vi "运维调试_总磷总氮.vi"() -> ()   [LabVIEW 2016, in "斯坦道总氮.lvlib"]
uses:
  <vilib>/Utility/miscctls.llb/LVPointTypeDef.ctl
  <vilib>/Plasmionique/MB Master/MB_Master/MB_Master.lvclass
  <vilib>/ptbypt/NI_PtbyPt.lvlib
  Alarm interface/Alarm interface.lvlib
panel:
  in  "周期设置":bool
  in  "流程操作":bool
  out "消解压力":sgl format="%#.2f kPa"
  out "权限等级":string
  out "总步数":i32
  out "滑动杆":u8(slide) caption="测试进度" scale=0.0..100.0
  in  "关闭心跳包":bool
  out "试剂余量显示":sgl[][](graph)
  in  "仪器校准":bool
  in  "参数查询":bool
  out "简易步骤名称":string
  in  "温度曲线":bool
  in  "试剂余量":bool
  in  "灯值调整":bool
  out "固件版本号":string
  out "模块版本号":string
  out "注射器温度":sgl format="%#.2f ℃"
  out "消解温度":sgl format="%#.2f ℃"
  out "ADC":sgl
  out "F3":sgl format="%#.6f"
  out "F2":sgl format="%#.6f"
  out "F1":sgl format="%#.6f"
  out "F0":sgl format="%#.6f"
  out "运行状态":T1 {"数据时间:" format="%<%y/%m/%d %H:%M:%S>T"; "仪器时间:" format="%<%y/%m/%d %H:%M:%S>T"}
  in  "单选按钮":T2=enum."总氮"
  in  "布尔":bool
  in  "外设固件":bool
  out "字符串 2":string
  in  "数组":string[](array[string])
  in  "返回":bool
  in  "参数设置":bool
  out "集成报警信息":string
  in  "停止":bool
  in  "手动启动":bool
  in  "调试":bool
  out "多列列表框":i32(listbox)
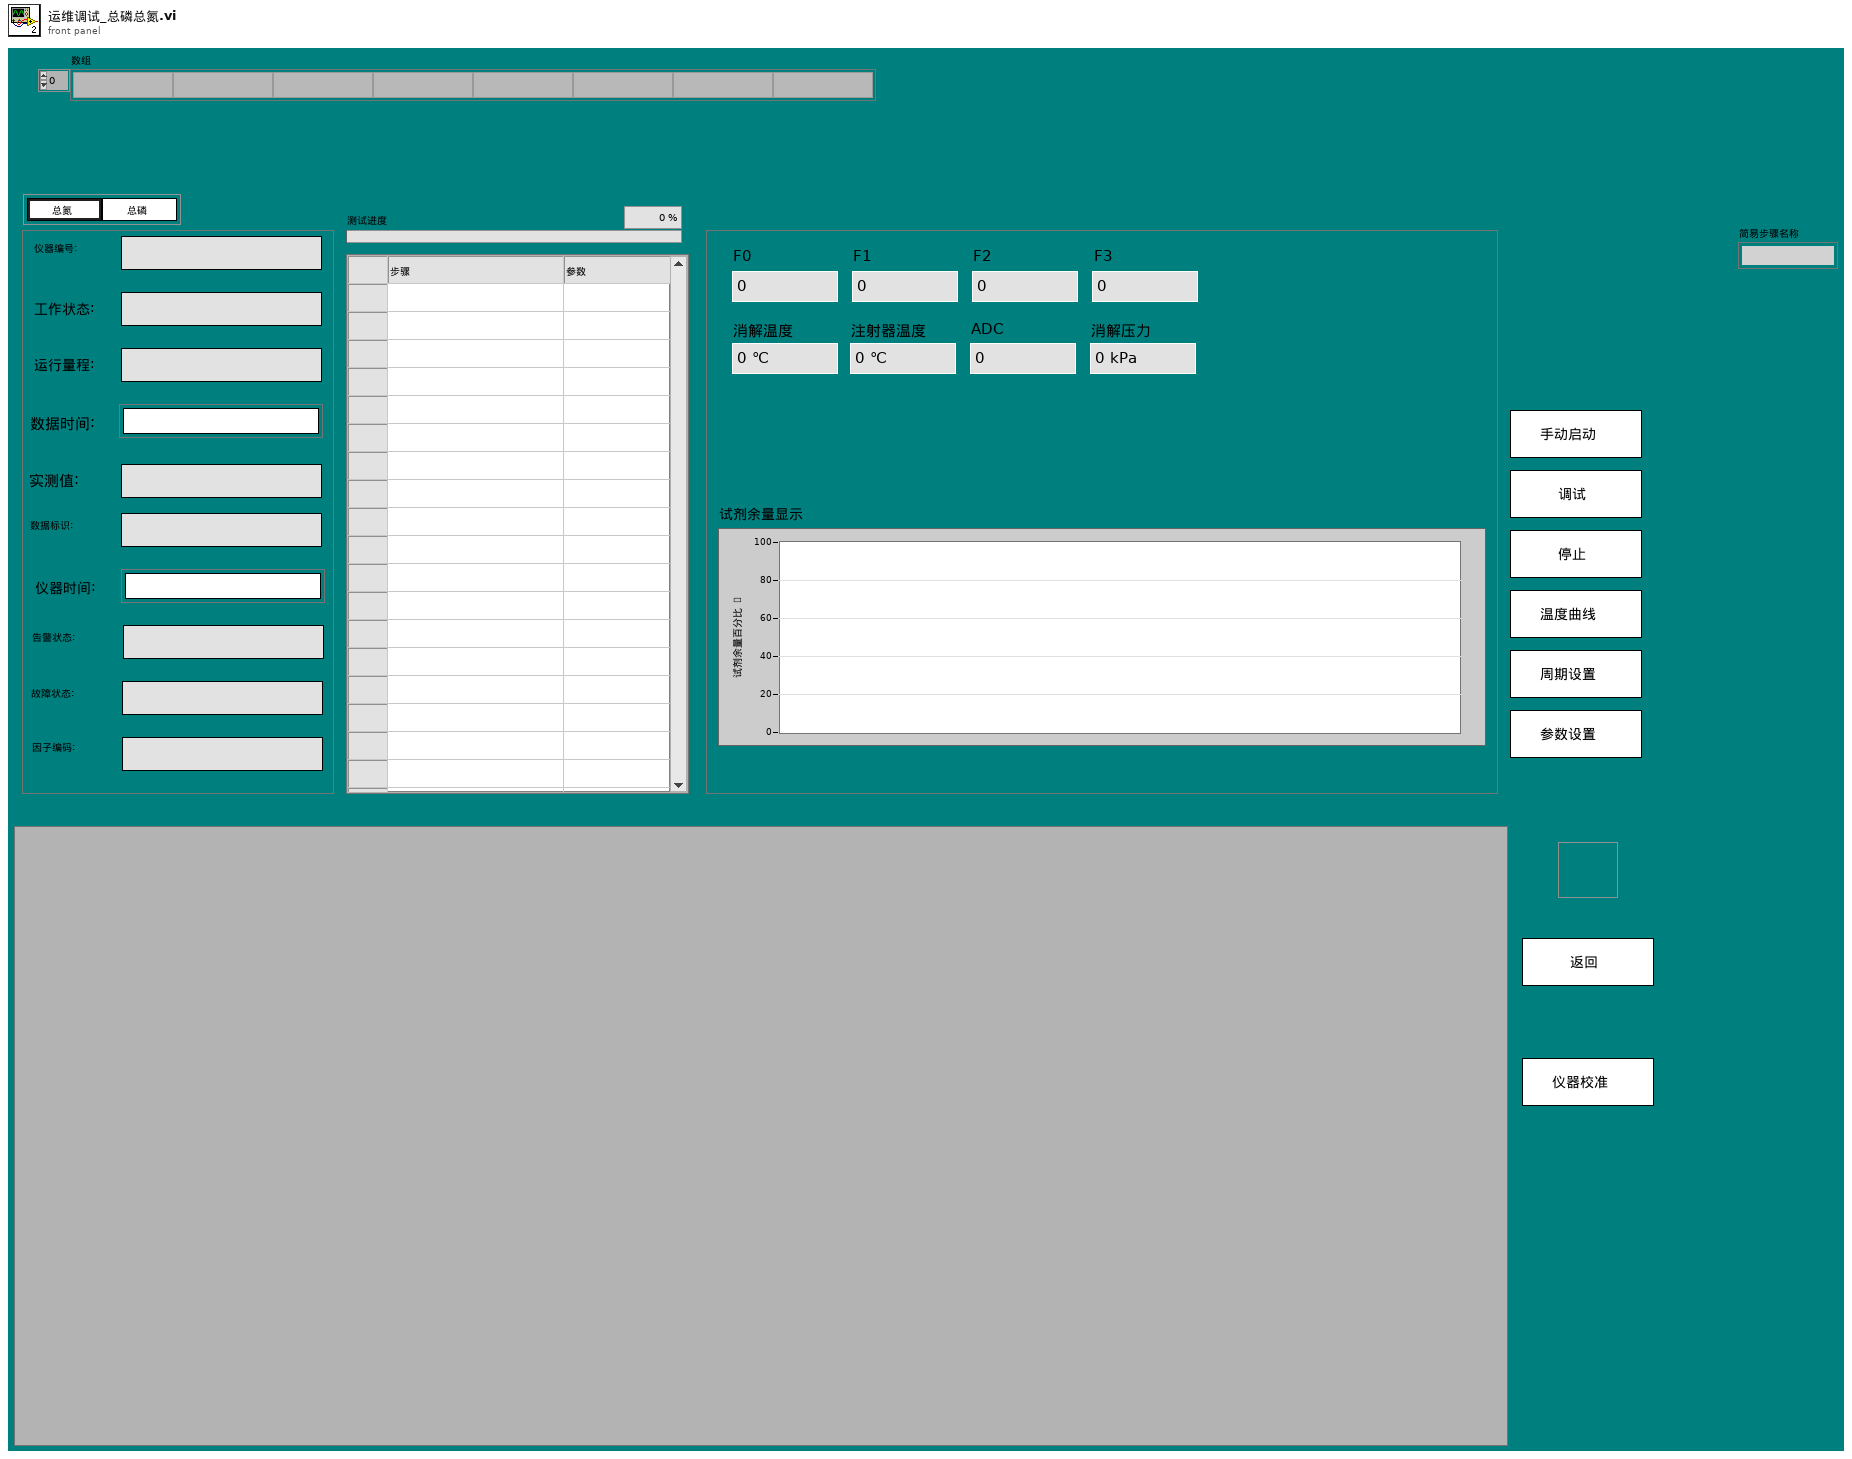
[diagram p1: front panel]
types:
  T1 = cluster{"仪器编号:":string, "工作状态:":string, "运行量程: ":string, "数据时间:":timestamp, "实测值:":string, "数据标识: ":string, "仪器时间:":timestamp, "告警状态: ":string, "故障状态:  ":string, "因子编码:":string}
  T2 = typedef "斯坦道总氮.lvlib/启动参数显示控件.ctl" = enum32{"COD", "氨氮", "总氮", "总磷", "磷酸盐", "硝氮", "亚硝氮", "硅酸盐", "硫化物", "氟化物"}
  T3 = cluster{"Major":u16, "Minor":u16, "Fix":u16, "Build":u16}
  T4 = enum32{"COD", "氨氮", "总氮", "总磷", "磷酸盐", "硝氮", "亚硝氮", "硅酸盐", "硫化物", "氟化物"}
  T5 = typedef "LVPointTypeDef.ctl" = cluster{"Horizontal":i16, "Vertical":i16}
  T6 = cluster{"系统时间":timestamp, "工作状态":u16, "测量模式":enum16{"待机", "连续模式", "周期模式", "定点模式", "受控模式", "手动模式"}, "告警代码":u16, "故障代码":u16, "日志代码":u16, "软件版本":u16, "F0":sgl, "F1":sgl, "F2":sgl, "F3":sgl, "T":sgl, "H":sgl, "id":u16, "flowid":u16, "量程":u16, "总磷控温温度1":sgl, "营养盐控温温度2":sgl, "ADC":sgl}
  T7 = cluster{"modid":i32, "sysid":i32, "content":string, "故障详情":string}
  T8 = typedef "SingleStepTestV3.lvlib/SingleStepTestV3.lvclass/仪器版本.ctl" = enum16{"A版", "B版"}
  T9 = cluster{"因子编码":u32, "单位":u16, "标样参考值":sgl, "水样数据时间":timestamp, "水样实测值":sgl, "水样数据标识":string, "标样数据时间":timestamp, "标样实测值":sgl, "标样数据标识":string, "空白数据时间":timestamp, "空白实测值":sgl, "空白数据标识":string, "零点核查数据时间":timestamp, "零点核查实测值":sgl, "零点核查数据标识":string, "跨度核查数据时间":timestamp, "跨度核查实测值":sgl, "跨度核查数据标识":string, "加标回收数据时间":timestamp, "加标回收实测值":sgl, "加标回收数据标识":string, "平行样数据时间":timestamp, "平行样实测值":sgl, "平行样数据标识":string, "F0":sgl, "F1":sgl, "F2":sgl, "F3":sgl, "F4":sgl, "F5":sgl, "F6":sgl, "F7":sgl, "温度":sgl, "湿度":sgl, "X值":sgl, "fidrange":u16, "X1值":sgl}[]
  T10 = cluster{"因子编码":u32, "单位":u16, "标样参考值":sgl, "水样数据时间":timestamp, "水样实测值":sgl, "水样数据标识":string, "标样数据时间":timestamp, "标样实测值":sgl, "标样数据标识":string, "空白数据时间":timestamp, "空白实测值":sgl, "空白数据标识":string, "零点核查数据时间":timestamp, "零点核查实测值":sgl, "零点核查数据标识":string, "跨度核查数据时间":timestamp, "跨度核查实测值":sgl, "跨度核查数据标识":string, "加标回收数据时间":timestamp, "加标回收实测值":sgl, "加标回收数据标识":string, "平行样数据时间":timestamp, "平行样实测值":sgl, "平行样数据标识":string, "F0":sgl, "F1":sgl, "F2":sgl, "F3":sgl, "F4":sgl, "F5":sgl, "F6":sgl, "F7":sgl, "温度":sgl, "湿度":sgl, "X值":sgl, "fidrange":u16, "X1值":sgl}
  T11 = typedef "报警信息字段定义.ctl" = cluster{"时间":timestamp, "参数":string, "报警信息":string, "备注":string, "code":u64}
  T12 = cluster{"module name":string, "moduleid":i32, "sysid":i32, "content":string, "analysis":string}
  T13 = cluster{"参数":string, "报警内容":string, "报警分析":string}
  T14 = typedef "TimingControl.lvlib/TimingControl.lvclass/国标控制命令.ctl" = enum16{"启动测量", "标样核查", "零点核查", "跨度核查", "空白测试", "平行样测试", "加标回收", "空白校准", "标样校准", "初始化（清洗）", "停止测试", "仪器重启", "校时", "模式设置", "测量间隔设置"}
  T15 = typedef "TimingControl.lvlib/TimingControl.lvclass/测量参数.ctl" = u16
  T16 = enum32{"Bad", "Idle", "Run top level", "Running"}
  T17 = enum16{"空闲", "水样测试", "标样核查", "零点核查", "跨度核查", "空白测试", "平行样测试", "加标回收", "空白校准", "标样校准", "初始化（清洗）"}
  T18 = cluster{"站号":u16, "量程切换":enum32{"H", "L", "AUTO"}, "控制命令":enum16{"启动测量", "标样核查", "零点核查", "跨度核查", "空白测试", "平行样测试", "加标回收", "空白校准", "标样校准", "初始化（清洗）", "停止测试", "仪器重启", "校时", "模式设置", "测量间隔设置"}, "模式设置":enum16{"待机", "连续模式", "周期模式", "定点模式", "受控模式", "手动模式"}, "测量间隔":u16}
  T19 = cluster{"时间标识":timestamp, "设备":string, "日志信息":string, "流程参数":string}
  T20 = typedef "LVRowAndColumnUnsignedTypeDef.ctl" = cluster{"Row":u32, "Column":u32}
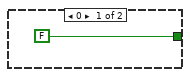
[diagram p4: hidden frame]
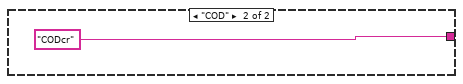
[diagram p5: hidden frame]
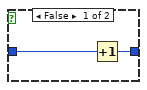
[diagram p7: hidden frame]
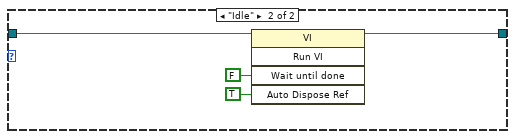
[diagram p8: hidden frame]
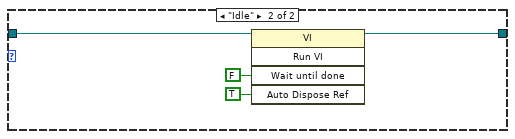
[diagram p9: hidden frame]
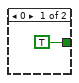
[diagram p11: hidden frame]
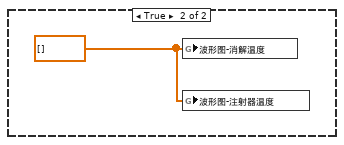
[diagram p12: hidden frame]
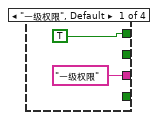
[diagram p16: hidden frame]
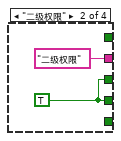
[diagram p17: hidden frame]
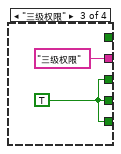
[diagram p18: hidden frame]
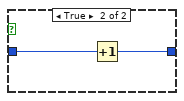
[diagram p20: hidden frame]
diagram:
  n1 = flat-sequence {
    tunnel: [w29] -> w20
    tunnel: [w31] -> w18
    tunnel: [w30] -> w2
    tunnel: w20 -> [w42]
    tunnel: [w42] -> w19
    tunnel: w18 -> [_]
    tunnel: w2 -> [_]
    tunnel: w19 -> [w65]
    tunnel: [w154] -> w21
    tunnel: [errorcluster {"status"=FALSE, "code"=0, "source"=""} ("错误输入（无错误）")] -> w9
    tunnel: [errorcluster {"status"=FALSE, "code"=0, "source"=""} ("错误输入（无错误）")] -> w8
    tunnel: [w151] -> w6
    tunnel: [errorcluster {"status"=FALSE, "code"=0, "source"=""} ("error out")] -> w5
    tunnel: [errorcluster {"status"=FALSE, "code"=0, "source"=""} ("错误输入（无错误）")] -> w4
    frame #0 {
      n2 = control-ref of="本VI"() -> (w32:refnum<vi>)
      n3 = control-ref of="本VI"() -> (w41:refnum<vi>)
      n4 = call "仪器配置读取.vi"() -> ("error out"=w31:errorcluster)  [unwired: 11 in]
      n5 = call "模块配置读取.vi"() -> ("error out"=w30:errorcluster)  [unwired: 11 in]
      n6 = property class="VI"(reference=w32) -> ("Library"=w33:refnum<vi>)  [unwired: 1 in, 2 out]
      n7 = property class="VI"(reference=w41) -> ("Library.Version"=w40:T3)  [unwired: 1 in, 2 out]
      n8 = property class="Library"(reference=w33) -> ("LocalName"=w29:string)  [unwired: 1 in, 2 out]
      n9 = Unbundle By Name(w40) -> ("Major"=w38:u16, "Minor"=w37:u16, "Fix"=w36:u16, "Build"=w35:u16)
      n10 = Format Into String(format string="模块版本号：%d.%d.%d.%d" ("格式字符串"), w38, w37, w36, w35) -> (resulting string=→"模块版本号":string)  [unwired: 2 in, 1 out]
    }
    frame #1 {
      n11 = global read "总磷总氮断电保存全局变量.vi" "IP"() -> (w46:string)
      n12 = global read "总磷总氮断电保存全局变量.vi" "VISA Resource"() -> (w43:refnum<visa-resource-name>)
      n13 = Empty String/Path?(string/path=w46) -> (empty?=w45:bool)
      n14 = Empty String/Path?(string/path=w43) -> (empty?=w44:bool)
      n15 = case shown="真" w45 {
        tunnel: w42 -> [_ w57]
        frame False {
        }
        frame True {
          n16 = case shown="\"斯坦道总氮.lvlib\"" w57 {
            tunnel: [w58 "192.168.1.203" ("IP") "192.168.1.202" ("IP") "192.168.1.202" ("IP") "192.168.1.203" ("IP") "192.168.1.204" ("IP") "192.168.1.205" ("IP")] -> w56
            frame Default {
              n17 = global read "总磷总氮断电保存全局变量.vi" "IP"() -> (w58:string)
            }
            frame "斯坦道总磷总氮.lvlib" {
            }
            frame "斯坦道氨氮.lvlib" {
            }
            frame "斯坦道氨氮总磷.lvlib" {
            }
            frame "斯坦道总磷.lvlib" {
            }
            frame "斯坦道总氮.lvlib" {
            }
            frame "斯坦道CODcr.lvlib" {
            }
          }
          n18 = global write "总磷总氮断电保存全局变量.vi" "IP"(w56) -> ()
        }
      }
      n19 = case shown="真" w44 {
        tunnel: w42 -> [_ w48]
        frame False {
        }
        frame True {
          n20 = case shown="\"斯坦道总氮.lvlib\"" w48 {
            tunnel: [w49 "COM5" ("IP") "COM7" ("IP") "COM7" ("IP") "COM5" ("IP") "COM10" ("IP") "COM9" ("IP")] -> w47
            frame Default {
              n21 = global read "总磷总氮断电保存全局变量.vi" "VISA Resource"() -> (w49:refnum<visa-resource-name>)
            }
            frame "斯坦道总磷总氮.lvlib" {
            }
            frame "斯坦道氨氮.lvlib" {
            }
            frame "斯坦道氨氮总磷.lvlib" {
            }
            frame "斯坦道总磷.lvlib" {
            }
            frame "斯坦道总氮.lvlib" {
            }
            frame "斯坦道CODcr.lvlib" {
            }
          }
          n22 = global write "总磷总氮断电保存全局变量.vi" "VISA Resource"(w47) -> ()
        }
      }
    }
    frame #2 {
      n23 = global read "model config var.vi" "启动队列名称"() -> (w67:cluster{"String":string, "Value":u16}[])
      n24 = Empty Array?(array=w67) -> (empty?=w66:bool)
      n25 = case shown="真" w66 {
        tunnel: w65 -> [_ w68]
        frame False {
        }
        frame True {
          n26 = global read "总磷总氮断电保存全局变量.vi" "PORT"() -> (w74:string)
          n27 = Decimal String To Number(string=w74) -> (number=w73:i32)  [unwired: 2 in, 1 out]
          n28 = global read "总磷总氮断电保存全局变量.vi" "MB通信方式选择"() -> (w72:enum16{"串口", "TCP"})
          n29 = global read "总磷总氮断电保存全局变量.vi" "VISA Resource"() -> (w71:refnum<visa-resource-name>)
          n30 = global read "总磷总氮断电保存全局变量.vi" "IP"() -> (w75:string)
          n31 = call "获取启动参数.vi"("MB通信方式选择"=w72, "Port (502)"=w73, "IP Address"=w75, "VISA Resource"=w71) -> ("error out"=w70:errorcluster, "数组"=w69:cluster{"String":string, "Value":u16}[])  [unwired: 6 in]
          n32 = flat-sequence {
            tunnel: w70 -> [w77]
            tunnel: w69 -> [w76]
            tunnel: w68 -> [w79]
            frame #0 {
              n33 = case shown="无错误" w77 {
                tunnel: w76 -> [w78 _]
                frame No Error {
                  n34 = global write "model config var.vi" "启动队列名称"(w78) -> ()
                }
                frame Error {
                }
              }
            }
            frame #1 {
              n35 = global read "model config var.vi" "启动队列名称"() -> (w81:cluster{"String":string, "Value":u16}[])
              n36 = Empty Array?(array=w81) -> (empty?=w80:bool)
              n37 = case shown="真" w80 {
                tunnel: w79 -> [_ w82]
                frame False {
                }
                frame True {
                  n38 = case shown="\"氟化物\"" w82 {
                    frame Default {
                    }
                    frame "斯坦道总磷总氮.lvlib" {
                      n39 = global write "model config var.vi" "启动队列名称"(cluster{"String":string, "Value":u16}[] [{"String"="总氮", "Value"=2}, {"String"="总磷", "Value"=1}] ("启动队列名称")) -> ()
                    }
                    frame "斯坦道氨氮.lvlib" {
                      n40 = global write "model config var.vi" "启动队列名称"(cluster{"String":string, "Value":u16}[] [{"String"="氨氮", "Value"=3}] ("启动队列名称")) -> ()
                    }
                    frame "斯坦道氨氮总磷.lvlib" {
                      n41 = global write "model config var.vi" "启动队列名称"(cluster{"String":string, "Value":u16}[] [{"String"="氨氮", "Value"=3}, {"String"="总磷", "Value"=1}] ("启动队列名称")) -> ()
                    }
                    frame "斯坦道总磷.lvlib" {
                      n42 = global write "model config var.vi" "启动队列名称"(cluster{"String":string, "Value":u16}[] [{"String"="总磷", "Value"=1}] ("启动队列名称")) -> ()
                    }
                    frame "斯坦道总氮.lvlib" {
                      n43 = global write "model config var.vi" "启动队列名称"(cluster{"String":string, "Value":u16}[] [{"String"="总氮", "Value"=2}] ("启动队列名称")) -> ()
                    }
                    frame "斯坦道CODcr.lvlib" {
                      n44 = global write "model config var.vi" "启动队列名称"(cluster{"String":string, "Value":u16}[] [{"String"="CODcr", "Value"=22}] ("启动队列名称")) -> ()
                    }
                    frame "氟化物" {
                      n45 = global write "model config var.vi" "启动队列名称"(cluster{"String":string, "Value":u16}[] [{"String"="氟化物", "Value"=50}] ("启动队列名称")) -> ()
                    }
                  }
                }
              }
            }
            frame #2 {
              n46 = call "模块配置写入.vi"() -> ()  [unwired: 11 in, 1 out]
            }
          }
        }
      }
    }
    frame #3 {
      # "初始化"
      n47 = flat-sequence {
        frame #0 {
          n48 = global read "总磷总氮断电保存全局变量.vi" "流程路径"() -> (w97:path)
          n49 = global read "总磷总氮断电保存全局变量.vi" "简易流程路径"() -> (w94:path)
          n50 = call <vilib>:"Check if File or Folder Exists.vi"("path"=w97) -> ("file or folder exists?"=w102:bool)  [unwired: 8 in, 2 out]
          n51 = call <vilib>:"Check if File or Folder Exists.vi"("path"=w94) -> ("file or folder exists?"=w101:bool)  [unwired: 8 in, 2 out]
          n52 = Empty String/Path?(string/path=w97) -> (empty?=w98:bool)
          n53 = Not(x=w102) -> (.not. x?=w100:bool)
          n54 = Empty String/Path?(string/path=w94) -> (empty?=w93:bool)
          n55 = Not(x=w101) -> (.not. x?=w96:bool)
          n56 = Or(x=w98, y=w100) -> (x .or. y?=w99:bool)
          n57 = Or(x=w93, y=w96) -> (x .or. y?=w95:bool)
          n58 = case shown="真" w99 {
            frame False {
            }
            frame True {
              n59 = global read "model config var.vi" "启动队列名称"() -> (w110:cluster{"String":string, "Value":u16}[])
              n60 = for {
                tunnel: w110 -> [w113] mode=indexing
                tunnel: [w112] -> w109 mode=indexing
                n61 = Unbundle By Name(w113) -> ("String"=w112:string)
              }
              n62 = call "获取默认流程路径.vi"("参数"=w109) -> ("路径"=w111:path)  [unwired: 10 in]
              n63 = global write "总磷总氮断电保存全局变量.vi" "流程路径"(w111) -> ()
            }
          }
          n64 = case shown="真" w95 {
            frame False {
            }
            frame True {
              n65 = global read "model config var.vi" "启动队列名称"() -> (w105:cluster{"String":string, "Value":u16}[])
              n66 = for {
                tunnel: w105 -> [w108] mode=indexing
                tunnel: [w107] -> w104 mode=indexing
                n67 = Unbundle By Name(w108) -> ("String"=w107:string)
              }
              n68 = call "获取默认流程路径.vi"("复合步骤"=TRUE, "参数"=w104) -> ("路径"=w106:path)  [unwired: 9 in]
              n69 = global write "总磷总氮断电保存全局变量.vi" "简易流程路径"(w106) -> ()
            }
          }
        }
        frame #1 {
          n70 = call "仪器配置写入.vi"() -> ()  [unwired: 11 in, 1 out]
        }
      }
      n71 = global read "model config var.vi" "启动队列名称"() -> (w90:cluster{"String":string, "Value":u16}[])
      n72 = for {
        tunnel: w90 -> [w117] mode=indexing
        shift-right: [w116] -> w91
        shift-left: "" -> [w114]
        n73 = Unbundle By Name(w117) -> ("String"=w115:string)
        n74 = Concatenate Strings(w114, w115) -> (w116:string)
      }
      n75 = global write "VAR总磷总氮全局变量.vi" "模块名称"(w91) -> ()
    }
    frame #4 {
      n76 = global read "model config var.vi" "启动队列名称"() -> (w120:cluster{"String":string, "Value":u16}[])
      n77 = vi-ref "总磷总氮测量数据储存.vi"() -> (w130:refnum<vi>)
      n78 = vi-ref "总磷总氮通讯.vi"() -> (w122:refnum<vi>)
      n79 = Index Array(array=w120) -> (element=w119:cluster{"String":string, "Value":u16})  [unwired: 1 in]
      n80 = property class="VI"(reference=w130) -> ("Name"=w137:string)  [unwired: 1 in, 2 out]
      n81 = property class="VI"(reference=w122) -> ("Name"=w123:string)  [unwired: 1 in, 2 out]
      n82 = Unbundle By Name(w119) -> ("Value"=w118:u16)
      n83 = case shown="50" w118 {
        tunnel: [w138 启动参数显示控件."总磷" ("单选按钮") 启动参数显示控件."总氮" ("单选按钮") 启动参数显示控件."COD" ("单选按钮") 启动参数显示控件."氨氮" ("单选按钮") 启动参数显示控件."磷酸盐" ("单选按钮") 启动参数显示控件."硝氮" ("单选按钮") 启动参数显示控件."亚硝氮" ("单选按钮") 启动参数显示控件."硅酸盐" ("单选按钮") 启动参数显示控件."硫化物" ("单选按钮") 启动参数显示控件."氟化物" ("单选按钮")] -> w121
        frame 0, Default {
          n84 = property on="单选按钮" class="RadioBtnsControl (严格)"() -> ("Value"=w138:T4)  [unwired: 2 in, 2 out]
        }
        frame 1 {
        }
        frame 2 {
        }
        frame 22 {
        }
        frame 3 {
        }
        frame 4 {
        }
        frame 5 {
        }
        frame 6 {
        }
        frame 7 {
        }
        frame 8 {
        }
        frame 50 {
        }
      }
      n85 = Open VI Reference(type specifier VI Refnum (for type only)=refnum<vi> refnum, vi path=w137, options=128 ("选项")) -> (vi reference=w135:refnum<vi>, error out=w133:errorcluster)  [unwired: 3 in]
      n86 = Open VI Reference(type specifier VI Refnum (for type only)=refnum<vi> refnum, vi path=w123, options=128 ("选项")) -> (vi reference=w125:refnum<vi>, error out=w127:errorcluster)  [unwired: 3 in]
      n87 = call-by-ref "开始异步调用"(reference=w135, error in=w133) -> (reference out=w131:refnum<vi>, error out=w132:errorcluster)  [unwired: 12 in]
      n88 = call-by-ref "开始异步调用"(reference=w125, error in=w127) -> (reference out=w129:refnum<vi>, error out=w128:errorcluster)  [unwired: 12 in]
      n89 = Close Reference(reference=w131, error in (no error)=w132) -> ()  [unwired: 1 out]
      n90 = Close Reference(reference=w129, error in (no error)=w128) -> ()  [unwired: 1 out]
      n91 = property on="单选按钮" class="RadioBtnsControl (严格)"("Value"=w121) -> ()  [unwired: 2 in, 2 out]
    }
    frame #5 {
      n92 = call "配置文件路径.vi"() -> ("appended path"=w151:path)  [unwired: 11 in]
      n93 = call "设置模块队列名.vi"() -> ("Msg"=w154:string)  [unwired: 5 in]
    }
  }
  n94 = flat-sequence {
    frame #0 {
      n95 = property on="窗格" class="Pane"("Origin"=T5 {"Horizontal"=0, "Vertical"=0} ("原点")) -> ()  [unwired: 2 in, 2 out]
    }
  }
  n96 = call "Create balloon 队列.vi"() -> ("队列输出"=w25:refnum<queue>)  [unwired: 11 in]
  n97 = while {
    stop <- FALSE stop-if-true
    n98 = global read "VAR总磷总氮全局变量.vi" "状态告警区"() -> (w160:T6)
    n99 = Unbundle By Name(w160) -> ("工作状态"=w158:u16)
    n100 = Equal To 0?(x=w158) -> (x = 0?=w157:bool)
    n101 = global read "VAR总磷总氮全局变量.vi" "通讯状态"() -> (w161:bool)
    n102 = And(x=w157, y=w161) -> (x .and. y?=w159:bool)
    n103 = call <vilib>:"Boolean Crossing PtByPt.vi"("input"=w159) -> ("crossing"=w156:bool)  [unwired: 2 in]
    n104 = case shown="真" w156 {
      frame False {
      }
      frame True {
        n105 = control-ref of="试剂余量显示"() -> (w164:refnum<vi>)
        n106 = call "试剂余量展示.vi"("波形图 2"=w164) -> ("波形图"=→"试剂余量显示":sgl[][])  [unwired: 10 in]
      }
    }
    n107 = Wait (ms)(milliseconds to wait=u32 1000 ("等待时间（毫秒）")) -> ()  [unwired: 1 out]
  }
  n108 = while {
    shift-right: [w176] -> _
    shift-left: u32 0 ("y") -> [w178]
    stop <- FALSE stop-if-true
    # "密码权限"
    n109 = global read "VAR总磷总氮全局变量.vi" "权限等级"() -> (w173:enum16{"一级权限", "二级权限", "三级权限", "超级权限"})
    n110 = case shown="\"超级权限\"" w173 {
      tunnel: [_ w183 w185 w188] -> w166
      tunnel: [_ _ w185 w188] -> _
      tunnel: [_ w183 w185 w188] -> w172
      tunnel: [_ _ _ TRUE] -> w171
      tunnel: [TRUE _ _ _] -> w169
      tunnel: ["一级权限" "二级权限" "三级权限" "超级权限"] -> w167
      frame "一级权限", Default {
      }
      frame "二级权限" {
        w183 = TRUE
      }
      frame "三级权限" {
        w185 = TRUE
      }
      frame "超级权限" {
        w188 = TRUE
      }
    }
    "权限等级" <- w167
    n111 = case shown="假" "布尔" {
      tunnel: w178 -> [_ w191]
      tunnel: [_ w190] -> w176
      frame False {
      }
      frame True {
        n112 = Increment(x=w191) -> (x+1=w190:u32)
      }
    }
    n113 = Wait (ms)(milliseconds to wait=u32 1000 ("等待时间（毫秒）")) -> ()  [unwired: 1 out]
    n114 = Not(x=w169) -> (.not. x?=w168:bool)
    n115 = property on="关闭心跳包" class="Bool (严格)"("Visible"=w171) -> ()  [unwired: 2 in, 2 out]
    n116 = property on="外设固件" class="Bool"("Visible"=w172) -> ()  [unwired: 2 in, 2 out]
    n117 = property on="流程操作" class="Bool"("Visible"=w166) -> ()  [unwired: 2 in, 2 out]
    n118 = property on="试剂余量" class="Bool"("Visible"=w166) -> ()  [unwired: 2 in, 2 out]
    n119 = property on="灯值调整" class="Bool"("Visible"=w166) -> ()  [unwired: 2 in, 2 out]
    n120 = Greater Or Equal?(x=w176, y=u32 3600) -> (x >= y?=w174:bool)
    n121 = property on="布尔" class="Bool (严格)"("Value"=w168) -> ()  [unwired: 2 in, 2 out]
    n122 = case shown="真" w174 {
      frame False {
      }
      frame True {
        n123 = global write "VAR总磷总氮全局变量.vi" "权限等级"(enum16{"一级权限", "二级权限", "三级权限", "超级权限"}."一级权限" ("权限等级")) -> ()
      }
    }
  }
  n124 = while {
    shift-right: [w202] -> _
    shift-left: u16 1 ("工作状态") -> [w200]
    stop <- FALSE stop-if-true
    (unwired) "注射器温度"
    n125 = global read "VAR总磷总氮全局变量.vi" "状态告警区"() -> (w223:T6)
    n126 = global read "VAR总磷总氮全局变量.vi" "通讯状态"() -> (w234:bool)
    n127 = global write "VAR总磷总氮全局变量.vi" "最近一次工作状态"(w200) -> ()
    n128 = global read "VAR总磷总氮全局变量.vi" "状态告警区"() -> (w232:T6)
    n129 = Unbundle By Name(w223) -> ("id"=w222:u16, "工作状态"=w218:u16)
    n130 = case shown="真" w234 {
      tunnel: ["通讯异常" ("集成报警信息") w340] -> w233
      frame False {
      }
      frame True {
        n131 = global read "VAR总磷总氮全局变量.vi" "状态告警区"() -> (w346:T6)
        n132 = Unbundle By Name(w346) -> ("工作状态"=w345:u16)
        n133 = feedback #1(0) -> (w343:i32)
        n134 = case shown="0" w345 {
          tunnel: w343 -> [_ w348]
          tunnel: [_ w347] -> w341
          frame 0 {
          }
          frame Default {
            n135 = Increment(x=w348) -> (x+1=w347:i32)
          }
        }
        n136 = feedback-in #1(w341) -> ()
        n137 = global read "VAR总磷总氮全局变量.vi" "测量状态"() -> (w339:string)
        n138 = Format Into String(format string="工作计时: %d 秒" ("格式字符串"), initial string=w339, w341) -> (resulting string=w340:string)  [unwired: 1 in, 1 out]
      }
    }
    "集成报警信息" <- w233
    n139 = Unbundle By Name(w232) -> ("flowid"=w199:u16, "系统时间"=w228:timestamp, "工作状态"=w227:u16, "告警代码"=w221:u16, "故障代码"=w220:u16, "量程"=w226:u16)
    n140 = case shown="\"氨氮\"" "单选按钮" {
      tunnel: [22 3 2 1 4 5 6 7 8 50] -> w203
      tunnel: [_ TRUE _ _ _ _ _ _ _ _] -> w194
      frame "COD", Default {
      }
      frame "氨氮" {
      }
      frame "总氮" {
      }
      frame "总磷" {
      }
      frame "磷酸盐" {
      }
      frame "硝氮" {
      }
      frame "亚硝氮" {
      }
      frame "硅酸盐" {
      }
      frame "硫化物" {
      }
      frame "氟化物" {
      }
    }
    n141 = case shown="1, 默认" w218 {
      tunnel: w222 -> [_ w289]
      frame 0 {
      }
      frame 1, Default {
        n142 = case shown="50" w289 {
          tunnel: [w290 启动参数显示控件."总磷" ("单选按钮") 启动参数显示控件."总氮" ("单选按钮") 启动参数显示控件."COD" ("单选按钮") 启动参数显示控件."氨氮" ("单选按钮") 启动参数显示控件."磷酸盐" ("单选按钮") 启动参数显示控件."硝氮" ("单选按钮") 启动参数显示控件."亚硝氮" ("单选按钮") 启动参数显示控件."硅酸盐" ("单选按钮") 启动参数显示控件."硫化物" ("单选按钮") 启动参数显示控件."氟化物" ("单选按钮")] -> w288
          frame 0, Default {
            n143 = property on="单选按钮" class="RadioBtnsControl (严格)"() -> ("Value"=w290:T4)  [unwired: 2 in, 2 out]
          }
          frame 1 {
          }
          frame 2 {
          }
          frame 22 {
          }
          frame 3 {
          }
          frame 4 {
          }
          frame 5 {
          }
          frame 6 {
          }
          frame 7 {
          }
          frame 8 {
          }
          frame 50 {
          }
        }
        n144 = property on="单选按钮" class="RadioBtnsControl (严格)"("Value"=w288) -> ()  [unwired: 2 in, 2 out]
      }
    }
    n145 = case shown="1" w227 {
      selector: w227 -> [w305 _ w311 w315 w318 w320 w322 w324 w326 w328 w330 w332 w334 w337]
      tunnel: [w306 "空闲" ("工作状态") "水样测量" ("工作状态") w314 "零点核查" ("工作状态") "跨度核查" ("工作状态") "空白测试" ("工作状态") "平行样测试" ("工作状态") "加标回收" ("工作状态") "空白校准" ("工作状态") "标样校准" ("工作状态") "初始化" ("工作状态") "单步调试" ("工作状态") w336] -> w201
      tunnel: [w304 w309 w311 w315 w318 w320 w322 w324 w326 w328 w330 w332 w334 w337] -> w202
      tunnel: w200 -> [w304 w309 _ _ _ _ _ _ _ _ _ _ _ _]
      tunnel: w199 -> [_ _ _ w313 _ _ _ _ _ _ _ _ _ _]
      frame Default {
        n146 = Format Into String(format string="%d" ("格式字符串"), initial string="未知" ("工作状态"), w305) -> (resulting string=w306:string)  [unwired: 1 in, 1 out]
      }
      frame 0 {
      }
      frame 1 {
      }
      frame 2 {
        n147 = case shown="5" w313 {
          tunnel: ["标样核查" ("工作状态") "快捷测试" ("工作状态")] -> w314
          frame 0, Default {
          }
          frame 5 {
          }
        }
      }
      frame 3 {
      }
      frame 4 {
      }
      frame 5 {
      }
      frame 6 {
      }
      frame 7 {
      }
      frame 8 {
      }
      frame 9 {
      }
      frame 10 {
      }
      frame 254 {
      }
      frame 255 {
        n148 = local read "简易步骤名称"() -> (w336:string)
      }
    }
    n149 = global read "VAR总磷总氮全局变量.vi" "模块名称"() -> (w192:string)
    n150 = case shown="1" w226 {
      tunnel: ["" ("字符串") "低量程 " ("字符串") "高量程 " ("字符串")] -> w225
      frame Default {
      }
      frame 0 {
      }
      frame 1 {
      }
    }
    n151 = call "告警码字段定义.vi"("模块名称"=w192, "告警代码"=w221) -> ("报警"=w198:T7)  [unwired: 9 in]
    n152 = Unbundle By Name(w198) -> ("content"=w197:string)
    n153 = call "id参数转换.vi"("id"=w203) -> ("数组资源索引"=w204:i32)  [unwired: 9 in, 1 out]
    n154 = call "版本判断.vi"() -> ("仪器版本"=w196:T8)  [unwired: 11 in]
    n155 = global read "VAR总磷总氮全局变量.vi" "测量数据区数组"() -> (w207:T9)
    n156 = case shown="\"A版\", 默认" w196 {
      tunnel: [w237 "传感器" ("标题.文本")] -> w193
      tunnel: ["%#.2f ℃" ("数值文本.格式字符串") "%#.2f " ("数值文本.格式字符串")] -> w195
      tunnel: w194 -> [w240 _]
      frame "A版", Default {
        n157 = Select(t="显色温度", s=w240, f="注射器温度" ("标题.文本")) -> (s? t:f=w237:string)
      }
      frame "B版" {
      }
    }
    n158 = Index Array(array=w207, index=w204) -> (element=w206:T10)
    n159 = case shown="0, 默认" w200 {
      tunnel: [w257 w263 w267 w271 w275 w279 w283 w287] -> w217
      tunnel: [w255 w262 w266 w270 w273 w278 w282 w286] -> w212
      tunnel: [w258 w261 w265 w269 w272 w277 w281 w285] -> w210
      tunnel: w206 -> [_ w260 w264 w268 w274 w276 w280 w284]
      frame 0, Default {
        n160 = local read "运行状态"() -> (w259:T1)
        n161 = Unbundle By Name(w259) -> ("数据时间:"=w257:timestamp, "实测值:"=w256:string, "数据标识:"=w258:string)
        n162 = Fract/Exp String To Number(string=w256) -> (number=w255:dbl)  [unwired: 3 in, 1 out]
      }
      frame 1 {
        n163 = Unbundle By Name(w260) -> ("水样数据时间"=w263:timestamp, "水样实测值"=w262:sgl, "水样数据标识"=w261:string)
      }
      frame 2, 9 {
        n164 = Unbundle By Name(w264) -> ("标样数据时间"=w267:timestamp, "标样实测值"=w266:sgl, "标样数据标识"=w265:string)
      }
      frame 3 {
        n165 = Unbundle By Name(w268) -> ("零点核查数据时间"=w271:timestamp, "零点核查实测值"=w270:sgl, "零点核查数据标识"=w269:string)
      }
      frame 4 {
        n166 = Unbundle By Name(w274) -> ("跨度核查数据时间"=w275:timestamp, "跨度核查实测值"=w273:sgl, "跨度核查数据标识"=w272:string)
      }
      frame 7 {
        n167 = Unbundle By Name(w276) -> ("加标回收数据时间"=w279:timestamp, "加标回收实测值"=w278:sgl, "加标回收数据标识"=w277:string)
      }
      frame 5, 8 {
        n168 = Unbundle By Name(w280) -> ("空白数据时间"=w283:timestamp, "空白实测值"=w282:sgl, "空白数据标识"=w281:string)
      }
      frame 6 {
        n169 = Unbundle By Name(w284) -> ("平行样数据时间"=w287:timestamp, "平行样实测值"=w286:sgl, "平行样数据标识"=w285:string)
      }
    }
    n170 = Unbundle By Name(w206) -> ("因子编码"=w208:u32)
    n171 = Wait (ms)(milliseconds to wait=u32 1000 ("等待时间（毫秒）")) -> ()  [unwired: 1 out]
    n172 = global write "VAR总磷总氮全局变量.vi" "工作状态:"(w201) -> ()
    n173 = Format Into String(format string="w%05d" ("格式字符串"), w208) -> (resulting string=w224:string)  [unwired: 2 in, 1 out]
    n174 = property on="注射器温度" class="DigNum (严格)"("Caption.Text"=w193, "NumText.FormatString"=w195) -> ()  [unwired: 2 in, 2 out]
    n175 = Number To Fractional String(number=w212, precision (6)=i16 4 ("精度(6)")) -> (F-format string=w214:string)  [unwired: 2 in]
    n176 = call "故障码字段定义.vi"("故障代码"=w220) -> ("字符串"=w219:string)  [unwired: 10 in]
    n177 = Concatenate Strings(w214, " " ("字符串"), "mg/L" ("字符串")) -> (w211:string)
    n178 = global read "VAR总磷总氮全局变量.vi" "序列号"() -> (w229:string)
    n179 = Bundle By Name(cluster=T1 {"仪器编号:"="", "工作状态:"="", "运行量程: "="", "数据时间:"=timestamp(0 s since 1904-01-01), "实测值:"="", "数据标识: "="", "仪器时间:"=timestamp(0 s since 1904-01-01), "告警状态: "="", "故障状态:  "="", "因子编码:"=""} ("运行状态"), "仪器编号:"=w229, "仪器时间:"=w228, "工作状态:"=w201, "告警状态:"=w197, "故障状态:"=w219, "运行量程:"=w225, "数据时间:"=w217, "实测值:"=w211, "数据标识:"=w210, "因子编码:"=w224) -> (→"运行状态":T1)
  }
  n180 = while {
    shift-right: [w353] -> _
    shift-left: 0 -> [w354]
    stop <- FALSE stop-if-true
    n181 = global read "VAR总磷总氮全局变量.vi" "心跳包打开状态"() -> (w349:bool)
    n182 = case shown="真" w349 {
      tunnel: w354 -> [w358 _]
      tunnel: [w357 _] -> w353
      frame False {
        n183 = Increment(x=w358) -> (x+1=w357:i32)
      }
      frame True {
      }
    }
    n184 = Wait (ms)(milliseconds to wait=u32 1000 ("等待时间（毫秒）")) -> ()  [unwired: 1 out]
    n185 = Greater Or Equal?(x=w353, y=3600) -> (x >= y?=w351:bool)
    n186 = case shown="真" w351 {
      frame False {
      }
      frame True {
        w356 = FALSE ("关闭心跳包")
        n187 = local write "关闭心跳包"(w356) -> ()
        n188 = global write "VAR总磷总氮全局变量.vi" "升级固件关闭心跳包"(w356) -> ()
      }
    }
  }
  n189 = while {
    shift-right: [w359] -> _
    shift-left: TRUE -> [w360]
    stop <- FALSE stop-if-true
    n190 = global read "VAR总磷总氮全局变量.vi" "状态告警区"() -> (w364:T6)
    n191 = global read "VAR总磷总氮全局变量.vi" "状态告警区"() -> (w367:T6)
    n192 = Unbundle By Name(w364) -> ("总磷控温温度1"=w363:sgl)
    n193 = Unbundle By Name(w367) -> ("工作状态"=w361:u16, "总磷控温温度1"=w366:sgl, "营养盐控温温度2"=w365:sgl)
    n194 = call "消解压力计算.vi"("当前消解温度"=w363) -> ("消解压力"=w362:dbl)  [unwired: 10 in]
    n195 = case shown="1, 默认" w361 {
      tunnel: w366 -> [_ w373]
      tunnel: w365 -> [_ w372]
      tunnel: w360 -> [_ w371]
      tunnel: [TRUE _] -> w359
      frame 0 {
      }
      frame 1, Default {
        n196 = case shown="假" w371 {
          tunnel: w373 -> [w379 _]
          tunnel: w372 -> [w378 _]
          frame False {
            n197 = global read "VAR总磷总氮全局变量.vi" "波形图-消解温度"() -> (w377:sgl[])
            n198 = global read "VAR总磷总氮全局变量.vi" "波形图-注射器温度"() -> (w376:sgl[])
            n199 = Build Array (concatenate)(w377, w379) -> (w375:sgl[])
            n200 = Build Array (concatenate)(w376, w378) -> (w374:sgl[])
            n201 = global write "VAR总磷总氮全局变量.vi" "波形图-消解温度"(w375) -> ()
            n202 = global write "VAR总磷总氮全局变量.vi" "波形图-注射器温度"(w374) -> ()
          }
          frame True {
            w380 = dbl[] [] ("波形图-消解温度")
            n203 = global write "VAR总磷总氮全局变量.vi" "波形图-消解温度"(w380) -> ()
            n204 = global write "VAR总磷总氮全局变量.vi" "波形图-注射器温度"(w380) -> ()
          }
        }
      }
    }
    n205 = property on="消解压力" class="DigNum (严格)"("Value"=w362) -> ()  [unwired: 2 in, 2 out]
    n206 = Wait (ms)(milliseconds to wait=u32 1000 ("等待时间（毫秒）")) -> ()  [unwired: 1 out]
  }
  n207 = while {
    tunnel: w25 -> [w387]
    shift-right: [w383] -> _
    shift-left: _ -> [w384]
    stop <- FALSE stop-if-true
    n208 = global read "VAR总磷总氮全局变量.vi" "状态告警区"() -> (w381:T6)
    n209 = Unbundle By Name(w381) -> ("工作状态"=w382:u16, "id"=w389:u16, "日志代码"=w388:u16, "故障代码"=w386:u16, "告警代码"=w385:u16)
    n210 = case shown="1, 默认" w382 {
      tunnel: w389 -> [_ _]
      tunnel: w388 -> [_ w401]
      tunnel: w387 -> [_ w400]
      tunnel: w386 -> [_ w399]
      tunnel: w385 -> [_ w398]
      tunnel: w384 -> [w392 w397]
      tunnel: [w392 w396] -> w383
      frame 0 {
      }
      frame 1, Default {
        n211 = Add(x=w399, y=w398) -> (x+y=w396:u16)
        n212 = Not Equal To 0?(x=w396) -> (x != 0?=w395:bool)
        n213 = Not Equal?(x=w396, y=w397) -> (x != y?=w394:bool)
        n214 = And(x=w395, y=w394) -> (x .and. y?=w393:bool)
        n215 = case shown="真" w393 {
          tunnel: w401 -> [_ w416]
          tunnel: w400 -> [_ w414]
          tunnel: w399 -> [_ w413]
          tunnel: w398 -> [_ w412]
          frame False {
          }
          frame True {
            n216 = global read "VAR总磷总氮全局变量.vi" "模块名称"() -> (w411:string)
            n217 = call "故障告警分析.vi"("告警代码"=w412, "故障代码"=w413, "运行步序"=w416, "参数"=w411) -> ("报警簇"=w410:T12, "报警内容"=w415:T13, "sysid"=w409:i32)  [unwired: 4 in, 1 out]
            n218 = Get Date/Time In Seconds() -> (seconds since 1Jan1904=w408:timestamp)
            n219 = Unbundle By Name(w415) -> ("参数"=w406:string, "报警内容"=w405:string, "报警分析"=w404:string)
            n220 = call "Alarm interface.vi"("簇"=w410) -> ()  [unwired: 10 in, 1 out]
            n221 = Bundle By Name(cluster=T11 {"时间"=timestamp(0 s since 1904-01-01), "参数"="", "报警信息"="", "备注"="", "code"=0} ("data in"), "时间"=w408, "参数"=w406, "报警信息"=w405, "备注"=w404, "code"=w409) -> (w407:T11)
            n222 = Bundle("报警内容"=w405, "报警分析"=w404) -> (w403:cluster{"报警内容":string, "报警分析":string})  [unwired: 1 in]
            n223 = call "总磷总氮报警信息.vi"("data in"=w407) -> ()  [unwired: 10 in, 1 out]
            n224 = call "balloon入队列.vi"("报警内容"=w403, "队列"=w414) -> ()  [unwired: 9 in, 1 out]
          }
        }
      }
    }
    n225 = Wait (ms)(milliseconds to wait=u32 100) -> ()  [unwired: 1 out]
  }
  n226 = while {
    shift-right: [w417] -> _
    shift-left: _ -> [w422]
    tunnel: w6 -> [w420]
    stop <- FALSE stop-if-true
    n227 = File/Directory Info(path=w420) -> (last mod=w417:timestamp, error out=w418:errorcluster)  [unwired: 1 in, 5 out]
    n228 = Not Equal?(x=w422, y=w417) -> (x != y?=w421:bool)
    n229 = case shown="真" w421 {
      tunnel: [_ w424] -> _
      tunnel: w418 -> [_ _]
      frame False {
      }
      frame True {
        n230 = call "仪器配置读取.vi"() -> ("error out"=w424:errorcluster)  [unwired: 11 in]
      }
    }
    n231 = Wait (ms)(milliseconds to wait=u32 1000 ("等待时间（毫秒）")) -> ()  [unwired: 1 out]
  }
  n232 = flat-sequence {
    tunnel: w5 -> [_]
    frame #0 {
      n233 = control-ref of="周期设置"() -> (w429:refnum<vi>)
      n234 = call "New TimingControl.vi"("Reference"=w429) -> ("error out"=w427:errorcluster, "TimingControl out"=w428:refnum<class "TimingControl.lvclass">)  [unwired: 9 in]
      n235 = call "taskqueue ref.vi"() -> ("队列输出"=w431:refnum<queue>)  [unwired: 10 in, 1 out]
      n236 = while {
        tunnel: w431 -> [w449]
        shift-right: [w445] -> _
        shift-left: u32 0 ("等待时间（毫秒）") -> [w443]
        shift-right: [w433] -> w426
        shift-left: w428 -> [w438]
        shift-right: [w432] -> w425
        shift-left: w427 -> [w437]
        stop <- FALSE stop-if-true
        n237 = global read "VAR总磷总氮全局变量.vi" "状态告警区"() -> (w451:T6)
        n238 = Unbundle By Name(w451) -> ("工作状态"=w448:u16, "系统时间"=w435:timestamp)
        n239 = Quotient & Remainder(x=w443, y=u32 30) -> (x-y*floor(x/y)=w441:u32)  [unwired: 1 out]
        n240 = Equal To 0?(x=w441) -> (x = 0?=w440:bool)
        n241 = case shown="1, 默认" w448 {
          tunnel: [FALSE TRUE] -> w434
          frame 0 {
          }
          frame 1, Default {
          }
        }
        n242 = Increment(x=w443) -> (x+1=w447:u32)
        n243 = Wait (ms)(milliseconds to wait=u32 500 ("等待时间（毫秒）")) -> ()  [unwired: 1 out]
        n244 = property class="TimingControl"(reference=w438, error in=w437, "Properties:仪器时间"=w435, "Properties:仪器运行状态"=w434) -> (reference out=w433:refnum<class "TimingControl.lvclass">, error out=w432:errorcluster, "Properties:命令输出"=w436:cluster{"启动":bool, "控制命令":T14, "测量参数":T15})
        n245 = Unbundle By Name(w436) -> ("启动"=w444:bool, "控制命令"=w450:T14)
        n246 = And(x=w444, y=w440) -> (x .and. y?=w439:bool)
        n247 = Select(t=w447, s=w444, f=u32 0 ("等待时间（毫秒）")) -> (s? t:f=w445:u32)
        n248 = case shown="真" w439 {
          tunnel: w450 -> [_ w455]
          tunnel: w449 -> [_ w458]
          frame False {
          }
          frame True {
            n249 = Get Queue Status(queue=w458) -> (queue out=w456:refnum<queue>, # elements in queue=w457:i32)  [unwired: 2 in, 6 out]
            n250 = Equal To 0?(x=w457) -> (x = 0?=w454:bool)
            n251 = case shown="真" w454 {
              tunnel: w456 -> [_ w460]
              tunnel: w455 -> [_ w459]
              frame False {
              }
              frame True {
                n252 = Enqueue Element(queue=w460, element=w459) -> ()  [unwired: 2 in, 3 out]
              }
            }
          }
        }
      }
      n253 = call "试剂余量后台任务.vi"() -> ()  [unwired: 12 in]
      n254 = call "task.vi"() -> ()  [unwired: 12 in]
      n255 = call "Close TimingControl.vi"("error in (no error)"=w425, "TimingControl in"=w426) -> ()  [unwired: 9 in, 1 out]
    }
  }
  n256 = while {
    tunnel: w5 -> [_]
    stop <- FALSE stop-if-true
    n257 = flat-sequence {
      frame #0 {
        n258 = global read "model config var.vi" "启动队列名称"() -> (w467:cluster{"String":string, "Value":u16}[])
        n259 = global read "model config var.vi" "启动队列名称"() -> (w465:cluster{"String":string, "Value":u16}[])
        n260 = for {
          tunnel: w467 -> [w473] mode=indexing
          shift-right: [w472] -> w468
          shift-left: "" -> [w470]
          n261 = Unbundle By Name(w473) -> ("String"=w471:string)
          n262 = Concatenate Strings(w470, w471) -> (w472:string)
        }
        n263 = for {
          tunnel: w465 -> [w475] mode=indexing
          tunnel: [w474] -> w466 mode=indexing
          n264 = Unbundle By Name(w475) -> ("String"=w474:string)
        }
        n265 = property on="单选按钮" class="RadioBtnsControl (严格)"() -> ("Controls[]"=w464:refnum<vi>[])  [unwired: 2 in, 2 out]
        n266 = global write "VAR总磷总氮全局变量.vi" "模块名称"(w468) -> ()
        n267 = for {
          tunnel: w464 -> [w483] mode=indexing
          tunnel: w466 -> [w482]
          n268 = property class="Ctl"(reference=w483) -> (reference out=w481:refnum<vi>, "Label.Text"=w477:string)  [unwired: 1 in, 1 out]
          n269 = case shown="默认" w477 {
            selector: w477 -> [w484 _]
            tunnel: [w484 "CODcr"] -> w476
            frame Default {
            }
            frame "COD" {
            }
          }
          n270 = Search 1D Array(1D array=w482, element=w476) -> (index of element=w480:i32)  [unwired: 1 in]
          n271 = Not Equal?(x=w480, y=-1) -> (x != y?=w478:bool)
          n272 = property class="Ctl"(reference=w481, "Visible"=w478) -> ()  [unwired: 1 in, 2 out]
        }
      }
      frame #1 {
        n273 = Wait (ms)(milliseconds to wait=u32 5000 ("等待时间（毫秒）")) -> ()  [unwired: 1 out]
      }
    }
  }
  n274 = vi-ref "校准设置页.vi"() -> (w13:refnum<vi>)
  n275 = vi-ref "参数设置页.vi"() -> (w17:refnum<vi>)
  n276 = call "时间延迟"("error in (no error)"=w4) -> ("error out"=w28:errorcluster)  [unwired: 10 in]
  n277 = Obtain Notifier(name (unnamed)=w21, notification data type=FALSE) -> (notifier out=w22:refnum<notifier>)  [unwired: 2 in, 2 out]
  n278 = Obtain Queue(name (unnamed)=w21, element data type=cluster{"命令":string, "data":variant} {"命令"="", "data"=variant}) -> (queue out=w24:refnum<queue>)  [unwired: 3 in, 2 out]
  n279 = property class="VI"(reference=w13, error in=w8) -> (reference out=w11:refnum<vi>, "Exec.State"=w12:T16)  [unwired: 1 out]
  n280 = property class="VI"(reference=w17, error in=w9) -> (reference out=w15:refnum<vi>, "Exec.State"=w16:T16)  [unwired: 1 out]
  n281 = while {
    tunnel: w24 -> [w500]
    stop <- FALSE stop-if-true
    n282 = global read "总磷总氮断电保存全局变量.vi" "MB通信方式选择"() -> (w498:enum16{"串口", "TCP"})
    n283 = Get Queue Status(queue=w500) -> (queue out=w499:refnum<queue>, # elements in queue=w495:i32)  [unwired: 2 in, 6 out]
    n284 = global read "VAR总磷总氮全局变量.vi" "MB session in"() -> (w496:refnum<class "MB_Master.lvclass">)
    n285 = global read "VAR总磷总氮全局变量.vi" "升级固件关闭心跳包"() -> (w490:bool)
    n286 = Not(x="关闭心跳包") -> (.not. x?=w492:bool)
    n287 = Not(x=w490) -> (.not. x?=w489:bool)
    n288 = case shown="\"串口\", 默认" w498 {
      tunnel: [w503 w504] -> w497
      frame "串口", Default {
        n289 = global read "总磷总氮断电保存全局变量.vi" "VISA Resource"() -> (w503:refnum<visa-resource-name>)
      }
      frame "TCP" {
        n290 = global read "总磷总氮断电保存全局变量.vi" "IP"() -> (w504:string)
      }
    }
    "字符串 2" <- w497
    n291 = property class="MB_Master"(reference=w496) -> ("Properties:Session Valid"=w494:bool)  [unwired: 1 in, 2 out]
    n292 = Compound Arithmetic op=AND ("复合运算")(w494, w492, w489) -> (w491:bool)
    n293 = Equal To 0?(x=w495) -> (x = 0?=w487:bool)
    n294 = global write "VAR总磷总氮全局变量.vi" "心跳包打开状态"(w491) -> ()
    n295 = And(x=w487, y=w491) -> (x .and. y?=w488:bool)
    n296 = case shown="真" w488 {
      tunnel: w499 -> [_ w527]
      frame False {
      }
      frame True {
        n297 = global read "VAR总磷总氮全局变量.vi" "状态告警区"() -> (w520:T6)
        n298 = global read "VAR总磷总氮全局变量.vi" "MB session in"() -> (w514:refnum<class "MB_Master.lvclass">)
        n299 = Unbundle By Name(w520) -> ("系统时间"=w507:timestamp, "工作状态"=w516:u16)
        n300 = property class="MB_Master"(reference=w514) -> ("Properties:Session Valid"=w512:bool)  [unwired: 1 in, 2 out]
        n301 = Get Date/Time In Seconds() -> (seconds since 1Jan1904=w526:timestamp)
        n302 = global read "VAR总磷总氮全局变量.vi" "通讯状态"() -> (w515:bool)
        n303 = case shown="真" w512 {
          tunnel: [_ w529] -> w511
          frame False {
          }
          frame True {
            n304 = global read "VAR总磷总氮全局变量.vi" "MB session in"() -> (w528:refnum<class "MB_Master.lvclass">)
            n305 = call "总磷总氮版本号读取.vi"("MB session in"=w528) -> ("error out"=w529:errorcluster, "固件版本号"=w530:string)  [unwired: 8 in, 1 out]
            "固件版本号" <- w530
            n306 = global write "VAR总磷总氮全局变量.vi" "固件版本号"(w530) -> ()
          }
        }
        n307 = Subtract(x=w526, y=w507) -> (x-y=w525:dbl)
        n308 = Not Equal?(x=w507, y=timestamp(0 s since 1904-01-01)) -> (x != y?=w505:bool)
        n309 = And(x=w512, y=w515) -> (x .and. y?=w513:bool)
        n310 = Absolute Value(x=w525) -> (abs(x)=w524:dbl)
        n311 = Greater Or Equal?(x=w524, y=120.0) -> (x >= y?=w522:bool)
        n312 = global read "VAR总磷总氮全局变量.vi" "通讯状态"() -> (w508:bool)
        n313 = Compound Arithmetic op=AND ("复合运算")(w522, w508, w505) -> (w517:bool)
        n314 = case shown="真" w513 {
          tunnel: [_ w531] -> w510
          tunnel: w511 -> [_ w532]
          frame False {
          }
          frame True {
            n315 = global read "VAR总磷总氮全局变量.vi" "MB session in"() -> (w534:refnum<class "MB_Master.lvclass">)
            n316 = call "序列号读取.vi"("Error in"=w532, "MB session in"=w534) -> ("error out"=w531:errorcluster, "序列号"=w533:string)  [unwired: 7 in, 1 out]
            n317 = global write "VAR总磷总氮全局变量.vi" "序列号"(w533) -> ()
          }
        }
        n318 = global read "model config var.vi" "启动队列名称"() -> (w518:cluster{"String":string, "Value":u16}[])
        n319 = Unbundle By Name(w510) -> ("status"=w509:bool)
        n320 = Not(x=w509) -> ()  [unwired: 1 out]
        n321 = for {
          tunnel: [w552] -> w519 mode=indexing
          tunnel: w518 -> [w553] mode=indexing
          tunnel: w510 -> [_]
          n322 = Unbundle By Name(w553) -> ("Value"=w552:u16)
        }
        n323 = for {
          tunnel: w516 -> [w538]
          shift-right: [w539] -> w521
          shift-left: w527 -> [w541]
          tunnel: w519 -> [w535] mode=indexing
          n324 = Equal?(x=w538, y=T17."空闲") -> (x = y?=w536:bool)
          n325 = Bundle By Name(cluster=cluster{"命令":string, "data":variant} {"命令"="", "data"=variant} ("元素"), "命令"="读状态告警区", "data"=w535) -> (w543:cluster{"命令":string, "data":variant})
          n326 = Enqueue Element(queue=w541, element=w543) -> (queue out=w540:refnum<queue>)  [unwired: 2 in, 2 out]
          n327 = case shown="真" w536 {
            tunnel: w540 -> [w545 w548]
            tunnel: w535 -> [_ w547]
            tunnel: [w545 w546] -> w539
            frame False {
            }
            frame True {
              n328 = Bundle By Name(cluster=cluster{"命令":string, "data":variant} {"命令"="", "data"=variant} ("元素"), "命令"="读测量数据区", "data"=w547) -> (w550:cluster{"命令":string, "data":variant})
              n329 = Enqueue Element(queue=w548, element=w550) -> (queue out=w546:refnum<queue>)  [unwired: 2 in, 2 out]
            }
          }
        }
        n330 = case shown="真" w517 {
          tunnel: w521 -> [_ w555]
          frame False {
          }
          frame True {
            n331 = call "总磷总氮启动命令.vi"("参数"=T18 {"站号"=3, "量程切换"=enum."AUTO", "控制命令"=enum."校时", "模式设置"=enum."待机", "测量间隔"=0}) -> ("启动命令"=w554:cluster{"命令":string, "data":variant})  [unwired: 10 in]
            n332 = Enqueue Element(queue=w555, element=w554) -> ()  [unwired: 2 in, 3 out]
          }
        }
      }
    }
    n333 = Wait (ms)(milliseconds to wait=u32 1000 ("等待时间（毫秒）")) -> ()  [unwired: 1 out]
  }
  n334 = while {
    tunnel: w28 -> [_]
    stop <- FALSE stop-if-true
    n335 = global read "VAR总磷总氮全局变量.vi" "状态告警区"() -> (w588:T6)
    n336 = global read "VAR总磷总氮全局变量.vi" "状态告警区"() -> (w586:T6)
    n337 = global read "VAR总磷总氮全局变量.vi" "状态告警区"() -> (w589:T6)
    n338 = global read "VAR总磷总氮全局变量.vi" "状态告警区"() -> (w590:T6)
    n339 = Unbundle By Name(w588) -> ("flowid"=w559:u16, "工作状态"=w578:u16, "id"=w579:u16)
    n340 = Unbundle By Name(w586) -> ("日志代码"=w585:u16)
    n341 = Unbundle By Name(w589) -> ("日志代码"=w562:u16)
    n342 = Unbundle By Name(w590) -> ("id"=w566:u16, "flowid"=w565:u16, "量程"=w564:u16, "工作状态"=w557:u16, "F0"=→"F0":sgl, "F1"=→"F1":sgl, "F2"=→"F2":sgl, "F3"=→"F3":sgl, "ADC"=→"ADC":sgl, "总磷控温温度1"=→"消解温度":sgl, "营养盐控温温度2"=→"注射器温度":sgl)
    n343 = Not Equal To 0?(x=w578) -> (x != 0?=w576:bool)
    n344 = case shown="0" w578 {
      frame 0 {
        n345 = local write "数组"(string[] [] ("数组")) -> ()
      }
      frame 1, Default {
      }
    }
    n346 = feedback #2(w585) -> (w587:u16)
    n347 = feedback-in #2(w585) -> ()
    n348 = feedback-in #3(w562) -> ()
    n349 = feedback #3(w562) -> (w592:u16)
    n350 = property on="总步数" class="DigNum (严格)"() -> ("Value"=w563:i32)  [unwired: 2 in, 2 out]
    n351 = Subtract(x=w562, y=1) -> (x-y=→"多列列表框":i32)
    n352 = Not Equal?(x=w585, y=w587) -> (x != y?=w584:bool)
    n353 = Not Equal?(x=w562, y=w592) -> (x != y?=w591:bool)
    n354 = Divide(x=w562, y=w563) -> (x/y=w561:dbl)
    n355 = Bundle("id"=w566, "flowid"=w565, "量程"=w564) -> (w567:cluster{"id":u16, "flowid":u16, "量程":u16})  [unwired: 1 in]
    n356 = call <vilib>:"Boolean Crossing PtByPt.vi"("direction"=enum16{"either", "false-true", "true-false"}."false-true", "input"=w576) -> ("crossing"=w580:bool)  [unwired: 1 in]
    n357 = call <vilib>:"Boolean Crossing PtByPt.vi"("direction"=enum16{"either", "false-true", "true-false"}."true-false", "input"=w576) -> ("crossing"=w575:bool)  [unwired: 1 in]
    n358 = case shown="真" w584 {
      frame False {
      }
      frame True {
        n359 = property on="多列列表框" class="MCListbox (严格)"() -> ("ItemNames"=w664:string[][], "Value"=w660:i32)  [unwired: 2 in, 2 out]
        n360 = Index Array(array=w664, index (row)=w660) -> (element=w663:string[])  [unwired: 1 in]
        n361 = Index Array(array=w663) -> (element=w662:string)  [unwired: 1 in]
        n362 = call "过滤筛选流程.vi"("字符串"=w662) -> ("匹配后偏移量"=w661:i32)  [unwired: 10 in]
        n363 = case shown="默认" w661 {
          tunnel: w662 -> [w666 _]
          tunnel: w660 -> [w665 _]
          frame Default {
            n364 = case shown="默认" w666 {
              selector: w666 -> [w672 w679]
              tunnel: [w672 w679] -> w668
              tunnel: [string[] [] ("数组") w674] -> w667
              tunnel: w665 -> [_ w678]
              frame "读数" {
              }
              frame Default {
                n365 = Equal?(x=w678, y=1) -> (x = y?=w676:bool)
                n366 = Select(t=string[] [], s=w676, f="数组") -> (s? t:f=w674:string[])
              }
            }
            n367 = for {
              N: 1 -> [_]
              tunnel: w668 -> [w681]
              shift-right: [w680] -> w669
              shift-left: w667 -> [w682]
              n368 = Search 1D Array(1D array=w682, element=w681) -> (index of element=w685:i32)  [unwired: 1 in]
              n369 = Format Into String(format string="%s" ("格式字符串"), w681) -> (resulting string=w686:string)  [unwired: 2 in, 1 out]
              n370 = Equal?(x=w685, y=-1) -> (x = y?=w683:bool)
              n371 = case shown="真" w683 {
                tunnel: w686 -> [_ w696]
                tunnel: w682 -> [w688 w700]
                tunnel: w681 -> [_ w699]
                tunnel: [w688 w698] -> w680
                frame False {
                }
                frame True {
                  n372 = global read "VAR总磷总氮全局变量.vi" "状态告警区"() -> (w695:T6)
                  n373 = global read "VAR总磷总氮全局变量.vi" "状态告警区"() -> (w710:T6)
                  n374 = global read "VAR总磷总氮全局变量.vi" "状态告警区"() -> (w713:T6)
                  n375 = Insert Into Array(array=w700, new element=w699) -> (w698:string[])  [unwired: 1 in]
                  n376 = Unbundle By Name(w695) -> ("工作状态"=w694:u16, "flowid"=w689:u16)
                  n377 = Unbundle By Name(w710) -> ("F0"=w707:sgl, "F1"=w706:sgl, "F2"=w705:sgl, "F3"=w704:sgl, "id"=w703:u16, "flowid"=w702:u16, "量程"=w701:u16)
                  n378 = Unbundle By Name(w713) -> ("id"=w691:u16)
                  n379 = case shown="2" w694 {
                    selector: w694 -> [w715 _ _ _ _ _ _ _ _ _ _ _]
                    tunnel: [w714 "【水样测试】" ("字符串") w718 "【零点核查】" ("字符串") "【跨度核查】" ("字符串") "【空白测试】" ("字符串") "【平行样测试】" ("字符串") "【加标回收】" ("字符串") "【空白校准】" ("字符串") "【标样校准】" ("字符串") "【单步调试】" ("字符串") w729] -> w692
                    tunnel: w689 -> [_ _ w717 _ _ _ _ _ _ _ _ _]
                    frame 0, Default {
                      n380 = Number To Decimal String(number=w715) -> (decimal integer string=w714:string)  [unwired: 1 in]
                    }
                    frame 1 {
                    }
                    frame 2 {
                      n381 = case shown="5" w717 {
                        tunnel: ["【标样核查】" ("字符串") "【快捷测试】" ("字符串")] -> w718
                        frame Default {
                        }
                        frame 5 {
                        }
                      }
                    }
                    frame 3 {
                    }
                    frame 4 {
                    }
                    frame 5 {
                    }
                    frame 6 {
                    }
                    frame 7 {
                    }
                    frame 8 {
                    }
                    frame 9 {
                    }
                    frame 254 {
                    }
                    frame 255 {
                      n382 = local read "简易步骤名称"() -> (w731:string)
                      n383 = Format Into String(format string="(%s)" ("格式字符串"), initial string="【简易流程】" ("工作状态"), w731) -> (resulting string=w729:string)  [unwired: 1 in, 1 out]
                    }
                  }
                  n384 = call "id参数转换.vi"("id"=w691) -> ("table输出"=w690:string)  [unwired: 9 in, 1 out]
                  n385 = Format Into String(format string="F0=%#f,F1=%#f,F2=%#f,F3=%#f,Flow=%d-%-d-%-d" ("格式字符串"), w707, w706, w705, w704, w703, w702, w701) -> (resulting string=w708:string)  [unwired: 2 in, 1 out]
                  n386 = Concatenate Strings(w692, w696) -> (w693:string)
                  n387 = Get Date/Time In Seconds() -> (seconds since 1Jan1904=w711:timestamp)
                  n388 = Bundle By Name(cluster=T19 {"时间标识"=timestamp(0 s since 1904-01-01), "设备"="", "日志信息"="", "流程参数"=""} ("data in"), "时间标识"=w711, "设备"=w690, "日志信息"=w693, "流程参数"=w708) -> (w712:T19)
                  n389 = call "总磷总氮操作日志.vi"("data in"=w712) -> ()  [unwired: 10 in, 1 out]
                }
              }
            }
            n390 = local write "数组"(w669) -> ()
          }
          frame -1 {
          }
        }
      }
    }
    n391 = case shown="真" w591 {
      tunnel: w562 -> [_ w766]
      frame False {
      }
      frame True {
        n392 = Subtract(x=w766, y=1) -> (x-y=w764:i32)
        n393 = Subtract(x=w764, y=5) -> (x-y=w768:i32)
        n394 = Greater Or Equal To 0?(x=w768) -> (x >= 0?=w767:bool)
        n395 = property on="多列列表框" class="MCListbox (严格)"() -> (error out=w772:errorcluster, "TopLeft"=w773:T20)  [unwired: 2 in, 1 out]
        n396 = Select(t=w768, s=w767, f=0) -> (s? t:f=w769:i32)
        n397 = Bundle By Name(cluster=w773, "Row"=w769) -> (w774:T20)
        n398 = property on="多列列表框" class="MCListbox (严格)"(error in=w772, "TopLeft"=w774) -> ()  [unwired: 1 in, 2 out]
      }
    }
    n399 = while {
      tunnel: w567 -> [w748]
      shift-right: [w744] -> _
      shift-left: _ -> [w745]
      shift-right: [w737] -> _
      shift-left: _ -> [w746]
      shift-right: [w738] -> _
      shift-left: _ -> [w743]
      shift-right: [w734] -> _
      shift-left: _ -> [w741]
      tunnel: w557 -> [w734]
      stop <- TRUE stop-if-true
      n400 = Not Equal?(x=w741, y=w734) -> (x != y?=w740:bool)
      n401 = case shown="255" w734 {
        tunnel: [w749 w750] -> w738
        frame 0, Default {
          n402 = global read "总磷总氮断电保存全局变量.vi" "流程路径"() -> (w749:path)
        }
        frame 255 {
          n403 = global read "总磷总氮断电保存全局变量.vi" "简易流程路径"() -> (w750:path)
        }
      }
      n404 = Not Equal To 0?(x=w734) -> (x != 0?=w733:bool)
      n405 = Not Equal?(x=w743, y=w738) -> (x != y?=w739:bool)
      n406 = Compound Arithmetic op=OR ("复合运算")(w739, w740) -> (w742:bool)
      n407 = And(x=w733, y=w742) -> (x .and. y?=w735:bool)
      n408 = case shown="真" w735 {
        tunnel: [w752 w762] -> w737
        tunnel: [w751 w761] -> w744
        tunnel: w748 -> [_ w756]
        tunnel: w746 -> [w752 _]
        tunnel: w745 -> [w751 _]
        tunnel: w738 -> [_ w755]
        tunnel: w734 -> [_ w754]
        frame False {
        }
        frame True {
          n409 = call "斯坦道XML解析.vi"("工作状态"=w754, "添加的路径"=w755, "参数簇"=w756) -> ("简易步骤名称"=→"简易步骤名称":string, "步骤时间"=w757:string[], "步骤名"=w759:string[])  [unwired: 6 in]
          n410 = for {
            tunnel: w759 -> [_] mode=indexing
            tunnel: [w763] -> w760 mode=indexing
            i -> [w763]
          }
          n411 = Build Array(w759, w757) -> (w758:string[][])
          n412 = Transpose 2D Array(2D array=w758) -> (transposed array=w761:string[][])
          n413 = Number To Decimal String(number=w760) -> (decimal integer string=w762:string[])  [unwired: 1 in]
        }
      }
      n414 = property on="多列列表框" class="MCListbox (严格)"("ItemNames"=w744, "RowHdrs[]"=w737) -> ()  [unwired: 2 in, 2 out]
      n415 = Array Size(array=w737) -> (size(s)=→"总步数":i32)
    }
    n416 = Multiply(x=w561, y=100.0) -> (x*y=w558:dbl)
    "滑动杆" <- w558
    n417 = case shown="真" w580 {
      tunnel: w578 -> [_ w637]
      tunnel: w579 -> [_ w634]
      tunnel: w559 -> [_ w632]
      frame False {
      }
      frame True {
        n418 = case shown="8" w637 {
          selector: w637 -> [w644 _ _ _ _ _ _ _ _ _ _ _]
          tunnel: [w643 "【水样测试】" ("字符串") w647 "【零点核查】" ("字符串") "【跨度核查】" ("字符串") "【空白测试】" ("字符串") "【平行样测试】" ("字符串") "【加标回收】" ("字符串") "【空白校准】" ("字符串") "【标样校准】" ("字符串") "【单步调试】" ("字符串") "【简易流程】" ("字符串")] -> w642
          tunnel: w632 -> [_ _ w646 _ _ _ _ _ _ _ _ _]
          frame 0, Default {
            n419 = Number To Decimal String(number=w644) -> (decimal integer string=w643:string)  [unwired: 1 in]
          }
          frame 1 {
          }
          frame 2 {
            n420 = case shown="5" w646 {
              tunnel: ["【标样核查】" ("字符串") "【快捷测试】" ("字符串")] -> w647
              frame 0, Default {
              }
              frame 5 {
              }
            }
          }
          frame 3 {
          }
          frame 4 {
          }
          frame 5 {
          }
          frame 6 {
          }
          frame 7 {
          }
          frame 8 {
          }
          frame 9 {
          }
          frame 254 {
          }
          frame 255 {
          }
        }
        n421 = call "id参数转换.vi"("id"=w634) -> ("table输出"=w633:string)  [unwired: 9 in, 1 out]
        n422 = Concatenate Strings("<<" ("字符串"), w642, "启动" ("字符串")) -> (w641:string)
        n423 = Get Date/Time In Seconds() -> (seconds since 1Jan1904=w639:timestamp)
        n424 = Bundle By Name(cluster=T19 {"时间标识"=timestamp(0 s since 1904-01-01), "设备"="", "日志信息"="", "流程参数"=""} ("data in"), "时间标识"=w639, "设备"=w633, "日志信息"=w641) -> (w638:T19)
        n425 = call "总磷总氮操作日志.vi"("data in"=w638) -> ()  [unwired: 10 in, 1 out]
      }
    }
    n426 = case shown="真" w575 {
      tunnel: w578 -> [_ w597]
      tunnel: w579 -> [_ w610]
      tunnel: w559 -> [_ w595]
      frame False {
      }
      frame True {
        n427 = case shown="2" w597 {
          selector: w597 -> [w617 _ _ _ _ _ _ _ _ _ _ _]
          tunnel: [w616 "【水样测试】" ("字符串") w620 "【零点核查】" ("字符串") "【跨度核查】" ("字符串") "【空白测试】" ("字符串") "【平行样测试】" ("字符串") "【加标回收】" ("字符串") "【空白校准】" ("字符串") "【标样校准】" ("字符串") "【单步调试】" ("字符串") "【简易流程】" ("字符串")] -> w598
          tunnel: w595 -> [_ _ w619 _ _ _ _ _ _ _ _ _]
          frame 0, Default {
            n428 = Number To Decimal String(number=w617) -> (decimal integer string=w616:string)  [unwired: 1 in]
          }
          frame 1 {
          }
          frame 2 {
            n429 = case shown="5" w619 {
              tunnel: ["【标样核查】" ("字符串") "【快捷测试】" ("字符串")] -> w620
              frame 0, Default {
              }
              frame 5 {
              }
            }
          }
          frame 3 {
          }
          frame 4 {
          }
          frame 5 {
          }
          frame 6 {
          }
          frame 7 {
          }
          frame 8 {
          }
          frame 9 {
          }
          frame 254 {
          }
          frame 255 {
          }
        }
        n430 = global read "VAR总磷总氮全局变量.vi" "状态告警区"() -> (w608:T6)
        n431 = call "id参数转换.vi"("id"=w610) -> ("table输出"=w609:string)  [unwired: 9 in, 1 out]
        n432 = Unbundle By Name(w608) -> ("F0"=w607:sgl, "F1"=w606:sgl, "F2"=w605:sgl, "F3"=w604:sgl, "id"=w603:u16, "flowid"=w602:u16, "量程"=w601:u16)
        n433 = Format Into String(format string="F0=%#f,F1=%#f,F2=%#f,F3=%#f,Flow=%d-%-d-%-d" ("格式字符串"), w607, w606, w605, w604, w603, w602, w601) -> (resulting string=w599:string)  [unwired: 2 in, 1 out]
        n434 = Concatenate Strings(w598, "停止" ("字符串"), ">>" ("字符串")) -> (w615:string)
        n435 = Get Date/Time In Seconds() -> (seconds since 1Jan1904=w613:timestamp)
        n436 = Bundle By Name(cluster=T19 {"时间标识"=timestamp(0 s since 1904-01-01), "设备"="", "日志信息"="", "流程参数"=""} ("data in"), "时间标识"=w613, "设备"=w609, "日志信息"=w615, "流程参数"=w599) -> (w612:T19)
        n437 = call "总磷总氮操作日志.vi"("data in"=w612) -> ()  [unwired: 10 in, 1 out]
      }
    }
    n438 = global write "VAR总磷总氮全局变量.vi" "测试进度"(w558) -> ()
    n439 = Wait (ms)(milliseconds to wait=u32 1000 ("等待时间（毫秒）")) -> ()  [unwired: 1 out]
  }
  n440 = case shown="\"Bad\", 默认" w12 {
    tunnel: w11 -> [w775 w779]
    tunnel: [w775 w776] -> w10
    frame "Bad", Default {
    }
    frame "Idle" {
      n441 = invoke class="VI" method="Run VI"(reference=w779, "Wait until done"=FALSE ("结束前等待"), "Auto Dispose Ref"=TRUE ("自动销毁引用")) -> (reference out=w776:refnum<vi>)  [unwired: 2 in, 4 out]
    }
  }
  n442 = case shown="\"Bad\", 默认" w16 {
    tunnel: w15 -> [w780 w784]
    tunnel: [w780 w781] -> w14
    frame "Bad", Default {
    }
    frame "Idle" {
      n443 = invoke class="VI" method="Run VI"(reference=w784, "Wait until done"=FALSE ("结束前等待"), "Auto Dispose Ref"=TRUE ("自动销毁引用")) -> (reference out=w781:refnum<vi>)  [unwired: 2 in, 4 out]
    }
  }
  n444 = while {
    tunnel: w24 -> [w788]
    tunnel: w22 -> [w787]
    tunnel: w14 -> [w786]
    tunnel: w10 -> [w785]
    stop <- FALSE stop-if-true
    n445 = event shown="[10] \"停止\": 值改变" {
      selector: _ -> [_ _ _ _ _ _ _ _ _ _ _ _ _ _]
      dyn-events: _ -> [_ _ _ _ _ _ _ _ _ _ _ _ _ _]
      timeout: _ -> [_ _ _ _ _ _ _ _ _ _ _ _ _ _]
      tunnel: w788 -> [_ _ _ _ _ _ _ _ w802 _ w813 _ _ _]
      tunnel: w787 -> [_ _ _ _ _ _ _ _ _ _ w812 _ _ _]
      tunnel: w786 -> [_ _ _ _ _ _ _ _ _ _ _ w817 _ _]
      tunnel: w785 -> [_ _ _ _ _ _ _ _ _ _ _ _ w823 _]
      event Timeout {
        n446 = event-data() -> ()  [unwired: 1 in, 3 out]
      }
      event "流程操作": Value Change {
        n447 = event-data() -> ()  [unwired: 1 in, 6 out]
        n448 = global read "总磷总氮断电保存全局变量.vi" "流程路径"() -> (w791:path)
        n449 = global read "总磷总氮断电保存全局变量.vi" "简易流程路径"() -> (w790:path)
        n450 = call "流程写入.vi"("简易流程路径"=w790, "添加的路径"=w791) -> ()  [unwired: 10 in]
      }
      event "温度曲线": Value Change {
        n451 = event-data() -> ()  [unwired: 1 in, 6 out]
        n452 = call "温度曲线显示.vi"() -> ()  [unwired: 12 in]
      }
      event "试剂余量": Value Change {
        n453 = event-data() -> ()  [unwired: 1 in, 6 out]
        n454 = call "试剂余量显示UI.vi"() -> ()  [unwired: 12 in]
      }
      event "灯值调整": Value Change {
        n455 = event-data() -> ()  [unwired: 1 in, 6 out]
        n456 = call "灯值调整对话框.vi"() -> ()  [unwired: 12 in]
      }
      event "布尔": Value Change {
        n457 = event-data() -> ("NewVal"=w792:bool)  [unwired: 1 in, 5 out]
        n458 = case shown="假" w792 {
          frame False {
            n459 = global write "VAR总磷总氮全局变量.vi" "权限等级"(enum16{"一级权限", "二级权限", "三级权限", "超级权限"}."一级权限" ("权限等级")) -> ()
          }
          frame True {
            n460 = global read "VAR总磷总氮全局变量.vi" "权限密码"() -> (w796:u32[])
            n461 = global read "VAR总磷总氮全局变量.vi" "权限等级"() -> (w794:enum16{"一级权限", "二级权限", "三级权限", "超级权限"})
            n462 = call "密码权限设置.vi"("权限输入"=w794, "权限密码"=w796) -> ("权限输出"=w795:enum16{"一级权限", "二级权限", "三级权限", "超级权限"})  [unwired: 9 in]
            n463 = global write "VAR总磷总氮全局变量.vi" "权限等级"(w795) -> ()
          }
        }
      }
      event "权限等级": Mouse Down {
        n464 = event-data() -> ()  [unwired: 1 in, 8 out]
        n465 = global read "VAR总磷总氮全局变量.vi" "权限密码"() -> (w799:u32[])
        n466 = global read "VAR总磷总氮全局变量.vi" "权限等级"() -> (w797:enum16{"一级权限", "二级权限", "三级权限", "超级权限"})
        n467 = call "密码权限设置.vi"("权限输入"=w797, "权限密码"=w799) -> ("权限输出"=w798:enum16{"一级权限", "二级权限", "三级权限", "超级权限"})  [unwired: 9 in]
        n468 = global write "VAR总磷总氮全局变量.vi" "权限等级"(w798) -> ()
      }
      event "外设固件": Value Change {
        n469 = event-data() -> ()  [unwired: 1 in, 6 out]
        n470 = call "流程固件设置对话框.vi"() -> ()  [unwired: 12 in]
      }
      event "手动启动": Value Change {
        n471 = event-data() -> ()  [unwired: 1 in, 6 out]
        n472 = call "总磷总氮启动参数对话框.vi"() -> ("确认"=w800:bool, "元素"=w801:cluster{"命令":string, "data":variant})  [unwired: 10 in]
        n473 = case shown="真" w800 {
          tunnel: w802 -> [_ w805]
          tunnel: w801 -> [_ w804]
          frame False {
          }
          frame True {
            n474 = Flush Queue(queue=w805) -> (queue out=w803:refnum<queue>)  [unwired: 1 in, 2 out]
            n475 = Enqueue Element(queue=w803, element=w804) -> ()  [unwired: 2 in, 3 out]
          }
        }
      }
      event "调试": Value Change {
        n476 = event-data() -> ()  [unwired: 1 in, 6 out]
        n477 = call "简易流程调试界面.vi"() -> ()  [unwired: 12 in]
      }
      event "停止": Value Change {
        n478 = event-data() -> ()  [unwired: 1 in, 6 out]
        n479 = global read "VAR总磷总氮全局变量.vi" "状态告警区"() -> (w807:T6)
        n480 = Send Notification(notification=TRUE ("通知"), notifier=w812) -> ()  [unwired: 1 in, 2 out]
        n481 = Unbundle By Name(w807) -> ("id"=w806:u16)
        n482 = Bundle By Name(cluster=T18 {"站号"=1, "量程切换"=enum."AUTO", "控制命令"=enum."停止测试", "模式设置"=enum."待机", "测量间隔"=0} ("参数"), "站号"=w806) -> (w808:T18)
        n483 = call "总磷总氮启动命令.vi"("参数"=w808) -> ("启动命令"=w809:cluster{"命令":string, "data":variant})  [unwired: 10 in]
        n484 = Enqueue Element(queue=w813, element=w809) -> ()  [unwired: 2 in, 3 out]
      }
      event "参数设置", "参数查询": Value Change {
        n485 = event-data() -> ()  [unwired: 1 in, 6 out]
        n486 = invoke on="子面板" class="SubPnl" method="Remove VI"() -> (error out=w818:errorcluster)  [unwired: 3 in, 2 out]
        n487 = global write "VAR总磷总氮全局变量.vi" "页面"(enum16{"主页", "参数页", "校准页"}."参数页" ("页面")) -> ()
        n488 = property on="仪器校准" class="Bool"("Visible"=TRUE ("可见")) -> ()  [unwired: 2 in, 2 out]
        n489 = property on="参数查询" class="Bool"("Visible"=FALSE ("可见")) -> ()  [unwired: 2 in, 2 out]
        n490 = invoke on="子面板" class="SubPnl" method="Insert VI"(error in=w818, "VI Ref"=w817) -> ()  [unwired: 2 in, 4 out]
        n491 = property on="窗格" class="Pane"("Origin"=T5 {"Horizontal"=0, "Vertical"=640} ("原点")) -> ()  [unwired: 2 in, 2 out]
      }
      event "仪器校准": Value Change {
        n492 = event-data() -> ()  [unwired: 1 in, 6 out]
        n493 = invoke on="子面板" class="SubPnl" method="Remove VI"() -> (error out=w824:errorcluster)  [unwired: 3 in, 2 out]
        n494 = property on="参数查询" class="Bool"("Visible"=TRUE ("可见")) -> ()  [unwired: 2 in, 2 out]
        n495 = property on="仪器校准" class="Bool"("Visible"=FALSE ("可见")) -> ()  [unwired: 2 in, 2 out]
        n496 = invoke on="子面板" class="SubPnl" method="Insert VI"(error in=w824, "VI Ref"=w823) -> ()  [unwired: 2 in, 4 out]
        n497 = global write "VAR总磷总氮全局变量.vi" "页面"(enum16{"主页", "参数页", "校准页"}."校准页" ("页面")) -> ()
      }
      event "返回": Value Change {
        n498 = event-data() -> ()  [unwired: 1 in, 6 out]
        n499 = global write "VAR总磷总氮全局变量.vi" "页面"(enum16{"主页", "参数页", "校准页"}."主页" ("页面")) -> ()
        n500 = property on="窗格" class="Pane"("Origin"=T5 {"Horizontal"=0, "Vertical"=0} ("原点")) -> ()  [unwired: 2 in, 2 out]
      }
    }
  }
